vi "this variable for joystick.vi"() -> ()   [LabVIEW 2017]
panel:
  in  "Stop Button":bool
  out "Variable1":bool
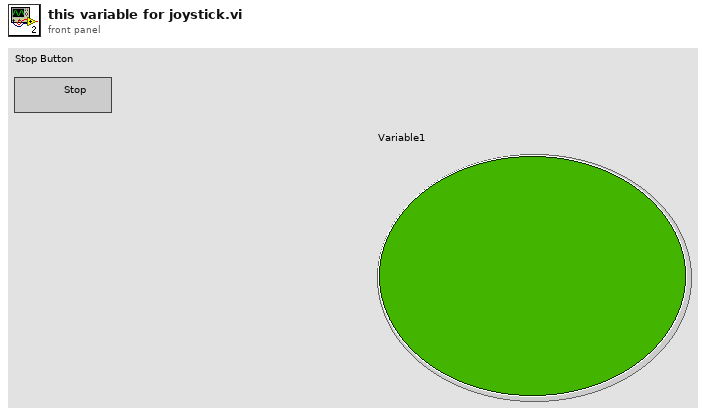
[diagram p1: front panel]
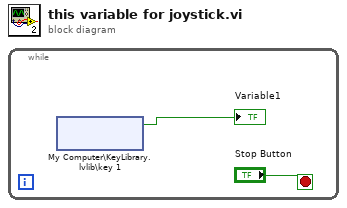
[diagram p0: block diagram]
diagram:
  n1 = while {
    stop <- "Stop Button" stop-if-true
    n2 = shared-variable "My Computer\\KeyLibrary.lvlib\\key 1"() -> (→"Variable1":bool)  [unwired: 1 in, 1 out]
  }
